vi "Command processing - 3 wheel omni.vi"(9 "Rotation scaling":dbl=0.5, 10 "Speed (0 to 1)":dbl=0.25, 11 "Command":T1(ring)) -> (0 "BR":dbl, 1 "BL":dbl, 3 "Top":dbl)   [LabVIEW 2016]
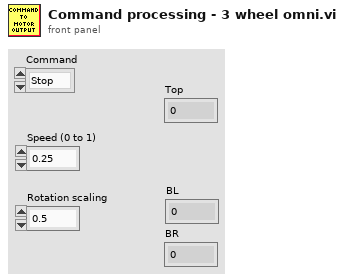
[diagram p1: front panel]
types:
  T1 = enum16{"Stop", "Forward", "Backward", "Left", "Right", "Clockwise", "Anticlockwise"}
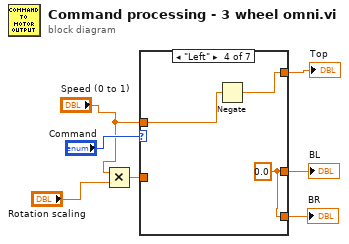
[diagram p0: block diagram]
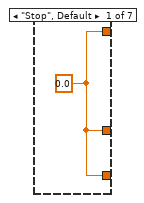
[diagram p2: hidden frame]
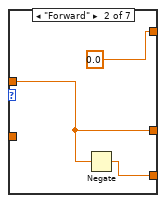
[diagram p3: hidden frame]
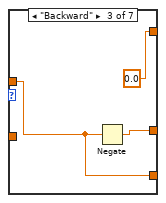
[diagram p4: hidden frame]
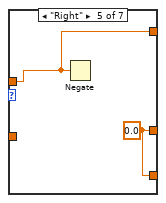
[diagram p5: hidden frame]
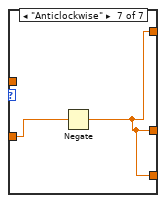
[diagram p7: hidden frame]
diagram:
  n1 = Multiply(x="Speed (0 to 1)", y="Rotation scaling") -> (x*y=w1:dbl)
  n2 = case shown="\"Left\"" "Command" {
    tunnel: [w8 0.0 ("Top") 0.0 ("Speed (-1 to 1)") w17 w19 w20 w21] -> w6
    tunnel: [w8 w10 w14 w15 w18 w20 w21] -> w5
    tunnel: [w8 w9 w13 w15 w18 w20 w21] -> w4
    tunnel: "Speed (0 to 1)" -> [_ w10 w13 w16 w19 _ _]
    tunnel: w1 -> [_ _ _ _ _ w20 w22]
    frame "Stop", Default {
      w8 = 0.0 ("Top")
    }
    frame "Forward" {
      n3 = Negate(x=w10) -> (-x=w9:dbl)
    }
    frame "Backward" {
      n4 = Negate(x=w13) -> (-x=w14:dbl)
    }
    frame "Left" {
      w15 = 0.0 ("Speed (-1 to 1)")
      n5 = Negate(x=w16) -> (-x=w17:dbl)
    }
    frame "Right" {
      w18 = 0.0 ("Speed (-1 to 1)")
      n6 = Negate(x=w19) -> ()  [unwired: 1 out]
    }
    frame "Clockwise" {
    }
    frame "Anticlockwise" {
      n7 = Negate(x=w22) -> (-x=w21:dbl)
    }
  }
  "Top" <- w6
  "BL" <- w5
  "BR" <- w4
